vi "SetPos.vi"(0 "Axis In":T4, 1 "Additional Settings":T1={"Next Index"=0, "Termination"=0, "Count"=1} {"Termination" items=["Stop", "Start Another Immediately", "Start Another x/start Index Input", "Start Another Index Without Stopping"]}, 5 "Index (0)":T3, 7 "Position":dbl, 11 "error in (no error)":errorcluster, 12 "Index Settings":T5={"Type"=1, "Dwell"=0, "Velocity"=0.0, "Accel/Decel"=0.0} {"Type" items=["Incremental", "Absolute", "Registration", "Jog"]}) -> (4 "Axis Out":T4, 6 "Index (duplicate)":T3, 15 "error out":errorcluster)   [LabVIEW 2009]
doc: "Send a position command to specified axis using the parameters in \"Index Settings\". Also saves this move to the index specified."
uses:
  typedefs/AxisSelect_Enum.ctl
  typedefs/Ultra3000/Index_Numeric.ctl
  typedefs/Ultra3000/IndexSettings_Cluster.ctl
  typedefs/Ultra3000/IndexType.ctl
  typedefs/DwellTime.ctl
  typedefs/Ultra3000/AdditionalIndexSettings_Cluster.ctl
  typedefs/Ultra3000/IndexTermination.ctl
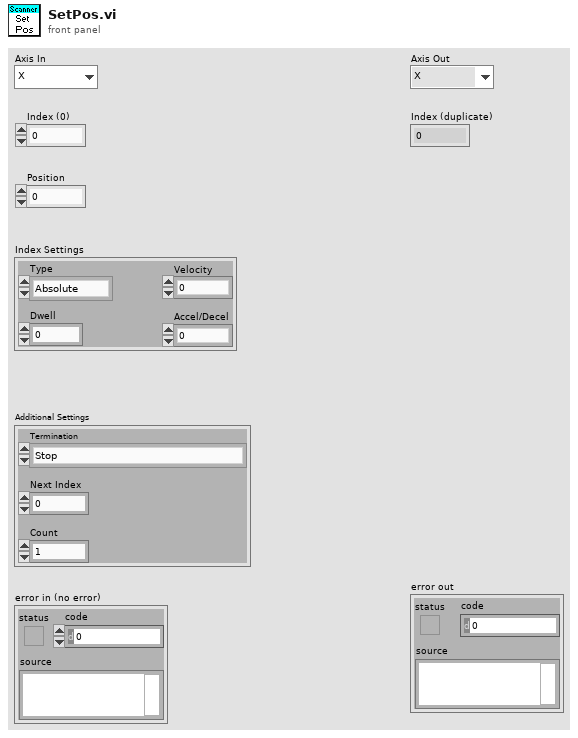
[diagram p1: front panel]
types:
  T1 = typedef "AdditionalIndexSettings_Cluster.ctl" = cluster{"Next Index":u8, "Termination":T2, "Count":u16}
  T2 = typedef "IndexTermination.ctl" = i32
  T3 = typedef "Index_Numeric.ctl" = u8
  T4 = typedef "AxisSelect_Enum.ctl" = enum16{"X", "Y", "Z", "Axis Space"}
  T5 = typedef "IndexSettings_Cluster.ctl" = cluster{"Type":T6, "Dwell":T7, "Velocity":dbl, "Accel/Decel":dbl}
  T6 = typedef "IndexType.ctl" = i32
  T7 = typedef "DwellTime.ctl" = u16
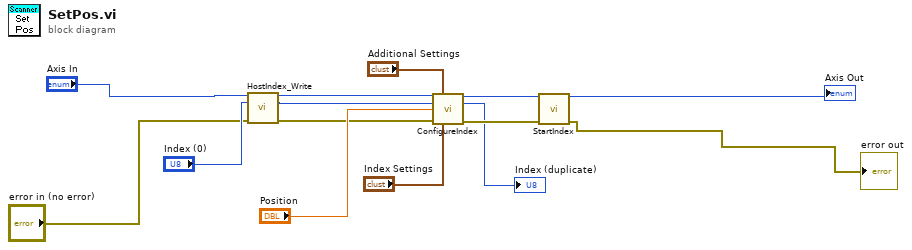
[diagram p0: block diagram]
diagram:
  n1 = call "HostIndex_Write.vi"("Axis In (Axis Space)"="Axis In", "Index"="Index (0)", "error in (no error)"="error in (no error)") -> ("Axis Out"=w5:T4, "Index (duplicate)"=w4:T3, "error out"=w1:errorcluster)  [unwired: 10 in]
  n2 = call "ConfigureIndex.vi"("Axis In"=w5, "Additional Settings"="Additional Settings", "Index (0)"=w4, "Position"="Position", "error in (no error)"=w1, "Index Settings"="Index Settings") -> ("Axis Out"=w12:T4, "Index (duplicate)"=→"Index (duplicate)":T3, "error out"=w10:errorcluster)  [unwired: 7 in]
  n3 = call "StartIndex.vi"("Axis In (Axis Space)"=w12, "error in (no error)"=w10) -> ("Axis Out"=→"Axis Out":T4, "error out"=→"error out":errorcluster)  [unwired: 12 in]
